vi "WPI_MotorControlDisable.vi"(8 "error in (no error)":errorcluster, 11 "MotorControlDevRef":T1={"DeviceStatus"={"status"=FALSE, "code"=0, "source"=""}, "Type"=enum."PWM", "PWM"={"PWM Channel"=enum."Invalid", "DeadBand"={"Name"="", "maxPositivePwm"=0, "minPositivePwm"=0, "centerPwm"=0, "maxNegativePwm"=0, "minNegativePwm"=0, "angularRange"=0}}, "CAN"={"Device Number"=0, "SetOutput VI Ref"=variant(enum8{"Percent VBus", "Current", "Speed", "Position", "Voltage"} enum."Percent VBus"), "GetOutput VI Ref"=variant(refnum<k1> refnum), "Enable VI Ref"=variant(dbl 12.0), "Disable VI Ref"=variant(enum8{"Percent VBus", "Speed", "Position", "Slave", "Unchanged / Invalid"} enum."Percent VBus"), "Data"=variant}, "Invert"=FALSE, "DIO PWM"={"PWM \"Enable\" Channel"=enum."Invalid", "DIOChannel"=enum."Invalid", "PWM Rate"=0.0}}) -> (0 "error out":errorcluster, 3 "MotorControlDevRef":T1={"DeviceStatus"={"status"=FALSE, "code"=0, "source"=""}, "Type"=enum."PWM", "PWM"={"PWM Channel"=enum."Invalid", "DeadBand"={"Name"="", "maxPositivePwm"=0, "minPositivePwm"=0, "centerPwm"=0, "maxNegativePwm"=0, "minNegativePwm"=0, "angularRange"=0}}, "CAN"={"Device Number"=0, "SetOutput VI Ref"=variant(enum8{"Percent VBus", "Current", "Speed", "Position", "Voltage"} enum."Percent VBus"), "GetOutput VI Ref"=variant(refnum<k1> refnum), "Enable VI Ref"=variant(dbl 12.0), "Disable VI Ref"=variant(enum8{"Percent VBus", "Speed", "Position", "Slave", "Unchanged / Invalid"} enum."Percent VBus"), "Data"=variant}, "Invert"=FALSE, "DIO PWM"={"PWM \"Enable\" Channel"=enum."Invalid", "DIOChannel"=enum."Invalid", "PWM Rate"=0.0}})   [LabVIEW 2017]
doc: "When the motor controller is connected via PWM, this VI will disable the PWM output on that channel. This is the same behavior that occurs with all PWM outputs in the event of a watchdog error. To resume output, simply call <B>SetOutput</B> again to set a new output VBus percentage.\n\nWhen the motor controller is connected via CAN, this VI will send a message to set output voltage to 0V and stop any running closed-loop controller on the motor controller. After calling this, you must call <B>Enable</B> to resume output and any closed-loop controller.\n\nThis software is licensed. Open the labview\\readme\\WPI Robotics Library Open Source License.txt file for more information."
uses:
  <vilib>/Rock Robotics/WPI/MotorControl/WPI_MotorControlDeviceRef.ctl
  <vilib>/Rock Robotics/WPI/MotorControl/WPI_MotorControlType.ctl
  <vilib>/Rock Robotics/SystemInterfaces/DIO/FPGA_DIOPWMChannel.ctl
  <vilib>/Rock Robotics/WPI/PWM/WPI_PWMDeadband.ctl
  <vilib>/Rock Robotics/SystemInterfaces/DIO/FPGA_DIOChannel.ctl
  <vilib>/Rock Robotics/WPI/PWM/WPI_PWMChannelCacheOp.ctl
  <vilib>/Rock Robotics/WPI/PWM/WPI_PWMSafetyCheck.vi
  <instrlib>/DC Motor Controller/HAIOL/DC Motor Controller.lvclass
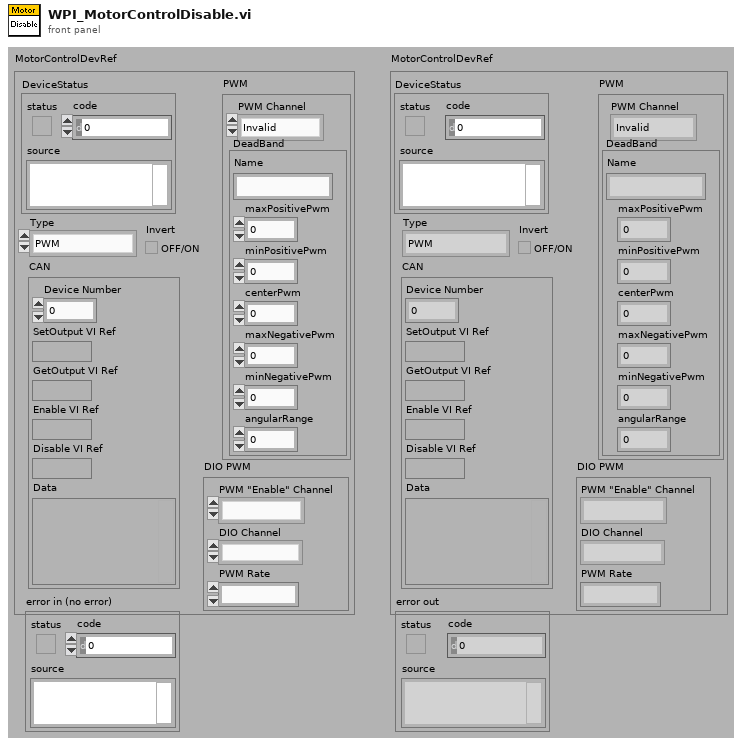
[diagram p1: front panel]
types:
  T1 = typedef "WPI_MotorControlDeviceRef.ctl" = cluster{"DeviceStatus":errorcluster, "Type":T2, "PWM":cluster{"PWM Channel":T3, "DeadBand":T4}, "CAN":cluster{"Device Number":u8, "SetOutput VI Ref":variant, "GetOutput VI Ref":variant, "Enable VI Ref":variant, "Disable VI Ref":variant, "Data":variant}, "Invert":bool, "DIO PWM":cluster{"PWM \"Enable\" Channel":T3, "DIOChannel":T5, "PWM Rate":dbl}}
  T2 = typedef "WPI_MotorControlType.ctl" = enum16{"PWM", "CAN", "DIO PWM"}
  T3 = typedef "FPGA_DIOPWMChannel.ctl" = enum8{"PWM 0", "PWM 1", "PWM 2", "PWM 3", "PWM 4", "PWM 5", "PWM 6", "PWM 7", "PWM 8", "PWM 9", "PWM MXP 0", "PWM MXP 1", "PWM MXP 2", "PWM MXP 3", "PWM MXP 4", "PWM MXP 5", "PWM MXP 6", "PWM MXP 7", "PWM MXP 8", "PWM MXP 9", "Invalid"}
  T4 = typedef "WPI_PWMDeadband.ctl" = cluster{"Name":string, "maxPositivePwm":i32, "minPositivePwm":i32, "centerPwm":i32, "maxNegativePwm":i32, "minNegativePwm":i32, "angularRange":u16}
  T5 = typedef "FPGA_DIOChannel.ctl" = enum8{"DIO 0", "DIO 1", "DIO 2", "DIO 3", "DIO 4", "DIO 5", "DIO 6", "DIO 7", "DIO 8", "DIO 9", "DIO MXP 0", "DIO MXP 1", "DIO MXP 2", "DIO MXP 3", "DIO MXP 4", "DIO MXP 5", "DIO MXP 6", "DIO MXP 7", "DIO MXP 8", "DIO MXP 9", "DIO MXP 10", "DIO MXP 11", "DIO MXP 12", "DIO MXP 13", "DIO MXP 14", "DIO MXP 15", "SPI Port CS1", "SPI Port CS2", "SPI Port CS3", "SPI Port MISO", "SPI Port MOSI", "Invalid"}
  T6 = typedef "WPI_PWMChannelCacheOp.ctl" = enum16{"Acquire", "Release", "Status"}
  T7 = typedef "WPI_PWMDeviceRef.ctl" = cluster{"DeviceStatus":errorcluster, "PWM Channel":T3}
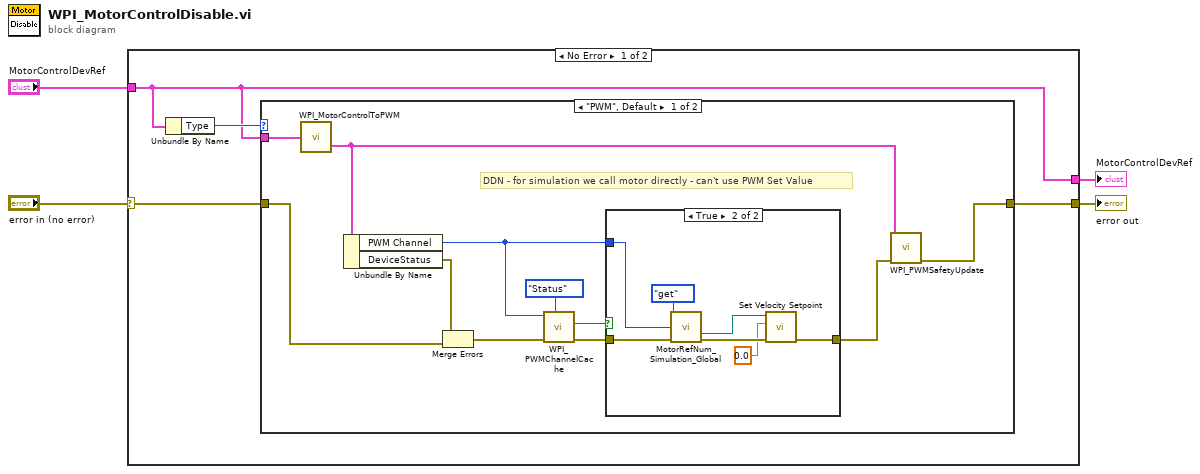
[diagram p0: block diagram]
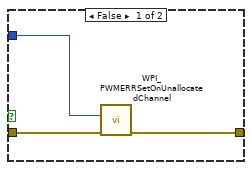
[diagram p2: hidden frame]
diagram:
  n1 = case shown="No Error" "error in (no error)" {
    selector: "error in (no error)" -> [w6 w32]
    tunnel: "MotorControlDevRef" -> [w5 w31]
    tunnel: [w5 w31] -> w1
    tunnel: [w8 w32] -> w2
    frame No Error {
      n2 = Unbundle By Name(w5) -> ("Type"=w7:T2)
      n3 = case shown="\"PWM\", Default" w7 {
        tunnel: w6 -> [w11 w30]
        tunnel: [w10 w30] -> w8
        tunnel: w5 -> [w19 _]
        frame "PWM", Default {
          # "DDN - for simulation we call motor directly - can't use PWM Set Value"
          n4 = call <vilib>:"WPI_MotorControlToPWM.vi"("MotorControlDeviceRef"=w19) -> ("PWMDeviceRef"=w9:T7)  [unwired: 1 out]
          n5 = Unbundle By Name(w9) -> ("PWM Channel"=w15:T3, "DeviceStatus"=w13:errorcluster)
          n6 = Merge Errors(w13, w11) -> (w14:errorcluster)
          n7 = call <vilib>:"WPI_PWMChannelCache.vi"("Operation"=WPI_PWMChannelCacheOp."Status", "error in (no error)"=w14, "PWMChannel"=w15) -> ("error out"=w17:errorcluster, "Allocated?"=w16:bool)  [unwired: 2 in, 5 out]
          n8 = case shown="True" w16 {
            tunnel: w17 -> [w22 w28]
            tunnel: [w21 w24] -> w18
            tunnel: w15 -> [w20 w26]
            frame False {
              n9 = call <vilib>:"WPI_PWMERRSetOnUnallocatedChannel.vi"("error in (no error)"=w22, "PWM Channel"=w20) -> ("error out"=w21:errorcluster)  [unwired: 9 in]
            }
            frame True {
              n10 = call <vilib>:"MotorRefNum_Simulation_Global.vi"("menu"=enum16{"set", "get", "delete"}."get", "PWM Channel"=w26, "error in (no error)"=w28) -> ("DC Motor Controller Get"=w25:refnum<class "DC Motor Controller.lvclass">, "error out"=w27:errorcluster)  [unwired: 11 in]
              n11 = call-dynamic "Set Velocity Setpoint.vi"("error in (no error)"=w27, "CCW Velocity (0 rad/s)"=0.0, "DC Motor Controller in"=w25) -> ("error out"=w24:errorcluster)  [unwired: 7 in, 1 out]
            }
          }
          n12 = call <vilib>:"WPI_PWMSafetyUpdate.vi"("error in (no error)"=w18, "PWMDeviceRef"=w9) -> ("error out"=w10:errorcluster)  [unwired: 9 out]
        }
        frame "CAN" {
        }
      }
    }
    frame Error {
    }
  }
  "MotorControlDevRef" <- w1
  "error out" <- w2
